vi "error_detail.vi"(10 "Error History 2":string, 11 "Device 2":string) -> ()   [LabVIEW 2020]
uses:
  Controls/comunicationQueuecluster.ctl
  Controls/PingQueueTypDef.ctl
  Controls/deviceQueue.ctl
  Controls/stopQue.ctl
  Controls/DeviceControl_Typdef.ctl
panel:
  in  "newDevice":bool=TRUE
  out "Device 3":string
  in  "Tab Control":enum32{"error", "Device", "GUI", "Computer"}(tab)=enum."Computer"
  out "Error History":string
  in  "start_device":bool=TRUE
  in  "restart_device":bool=TRUE
  in  "kill_device":bool=TRUE
  out "status:":string
  out "error:":string
  in  "Subscribed Variables":i32(listbox)
  out "response time":u32(slide) scale=0.0..5000.0
  out "devicetype:":string
  in  "start_GUI":bool=TRUE
  in  "rdp_PC":bool=TRUE
  in  "restart_PC":bool=TRUE
  out "IP":string
  in  "start_PC":bool
  in  "Cancel Button":bool
  in  "Device":bool
  in  "GUI":bool=TRUE
  in  "Computer":bool
  in  "Error":bool
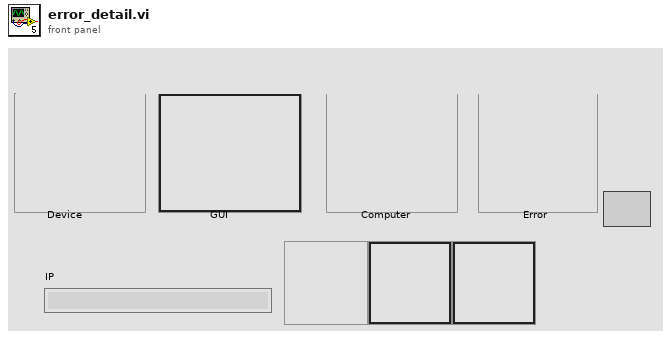
[diagram p1: front panel]
types:
  T1 = typedef "stopQue.ctl" = cluster{"stop":bool}
  T2 = enum8{"Enabled", "Disabled", "Disabled and Grayed Out"}
  T3 = typedef "deviceQueue.ctl" = cluster{"device":string[], "XY Graph":cluster{"x":u32[], "Ramp Pattern":dbl[]}, "ststus":string[], "error":string[], "error history":string[]}
  T4 = typedef "PingQueueTypDef.ctl" = cluster{"Computers not on":string[]}
  T5 = typedef "comunicationQueuecluster.ctl" = cluster{"device":string, "error history":string, "stop":bool}
  T6 = typedef "DeviceControl_Typdef.ctl" = enum16{"start", "stop", "kill", "PC rdp", "PC start", "PC shutdown", "PC restart", "GUI start"}
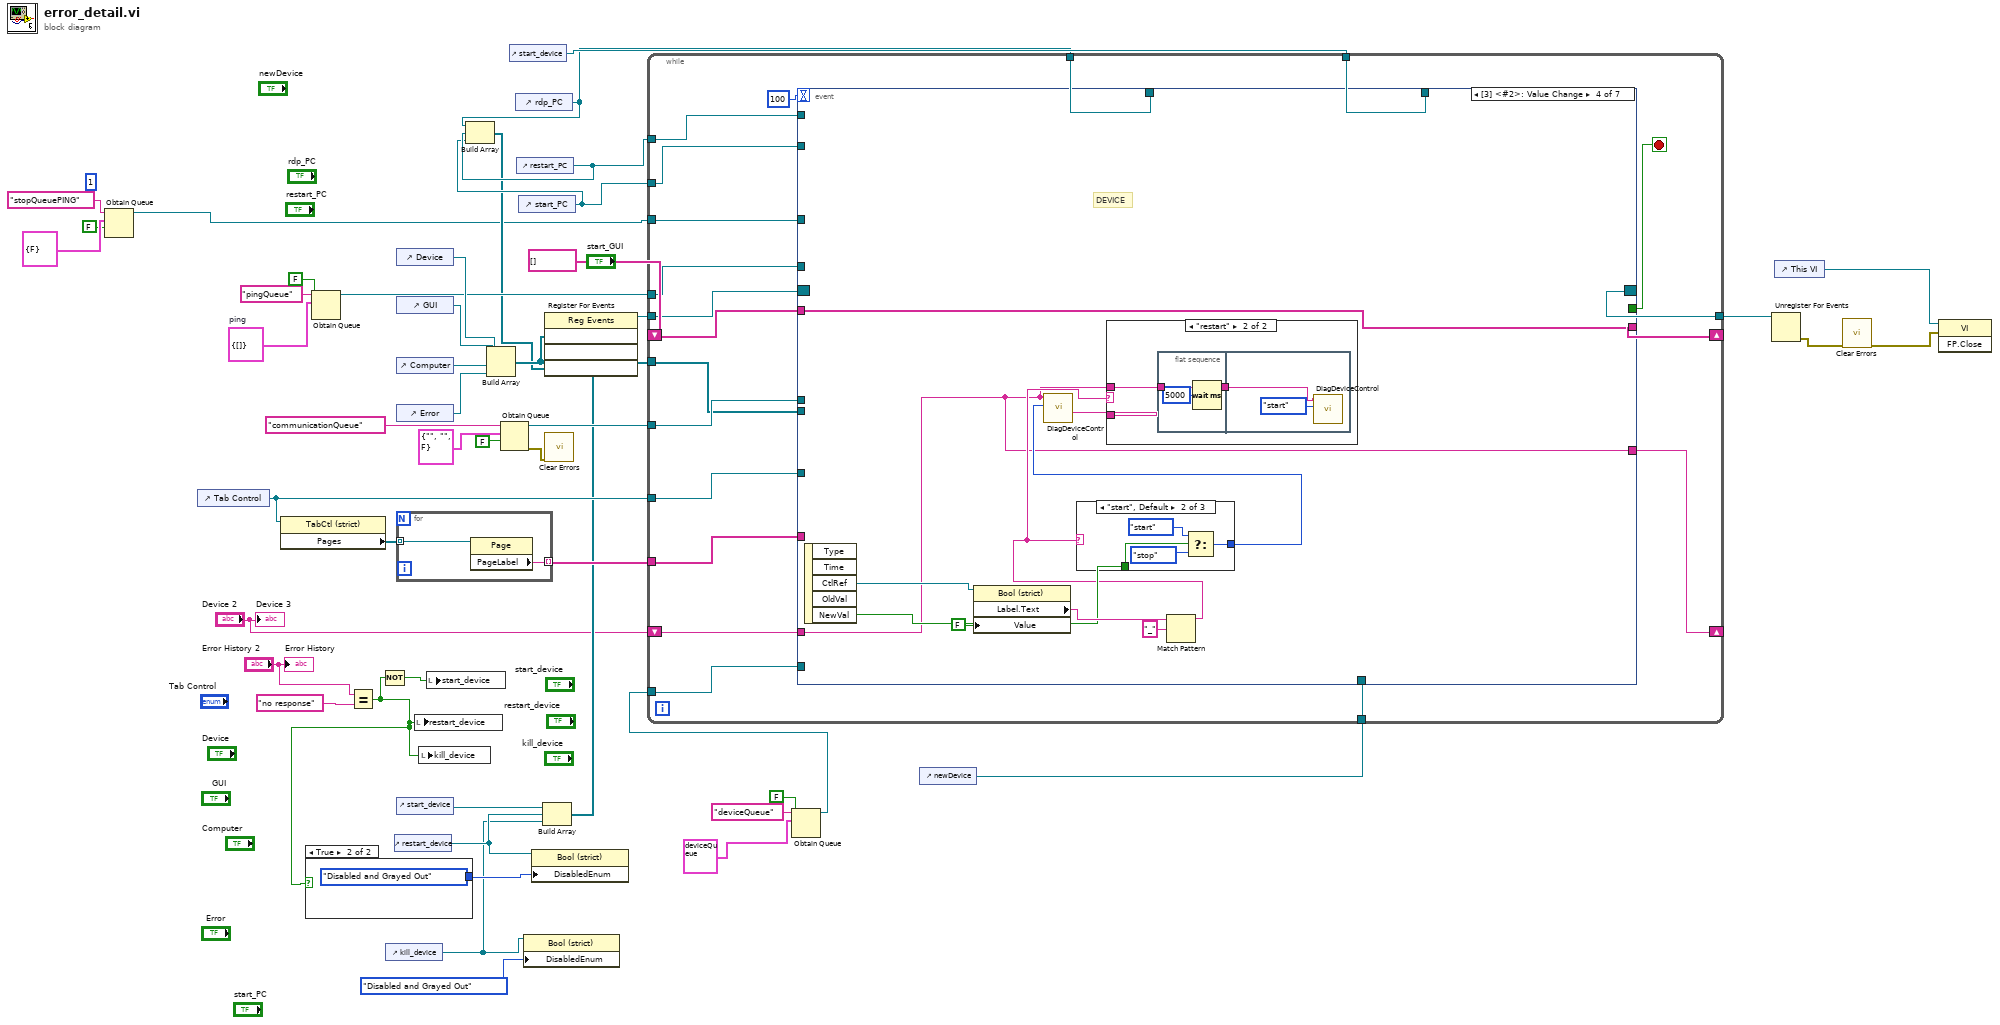
[diagram p0: block diagram]
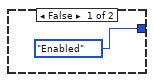
[diagram p2: hidden frame]
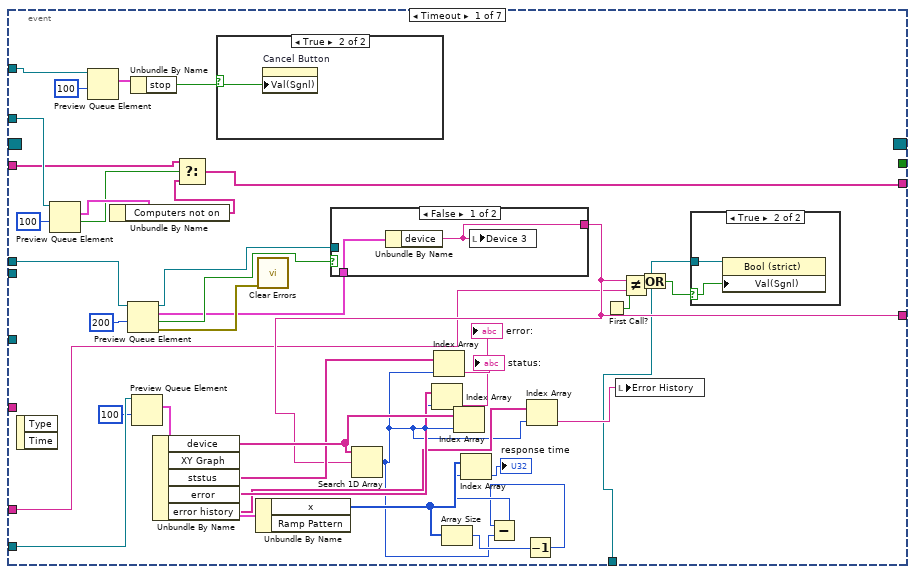
[diagram p3: hidden frame]
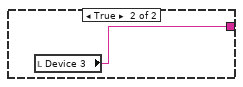
[diagram p6: hidden frame]
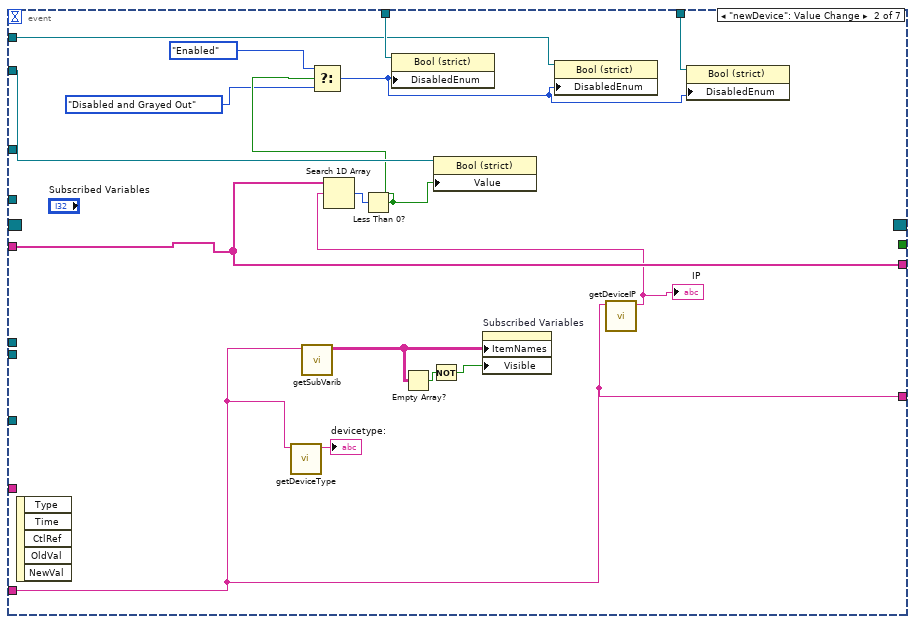
[diagram p7: hidden frame]
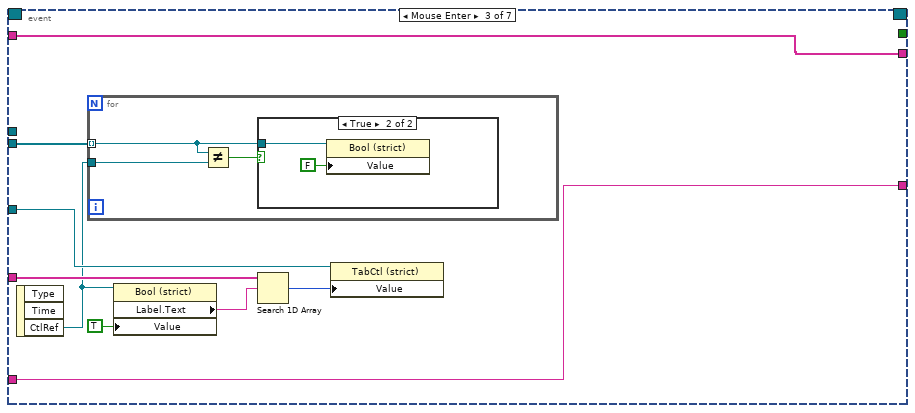
[diagram p8: hidden frame]
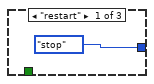
[diagram p11: hidden frame]
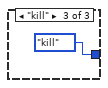
[diagram p12: hidden frame]
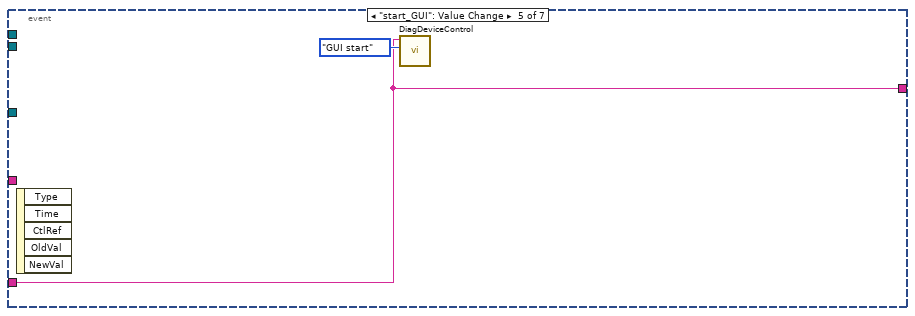
[diagram p13: hidden frame]
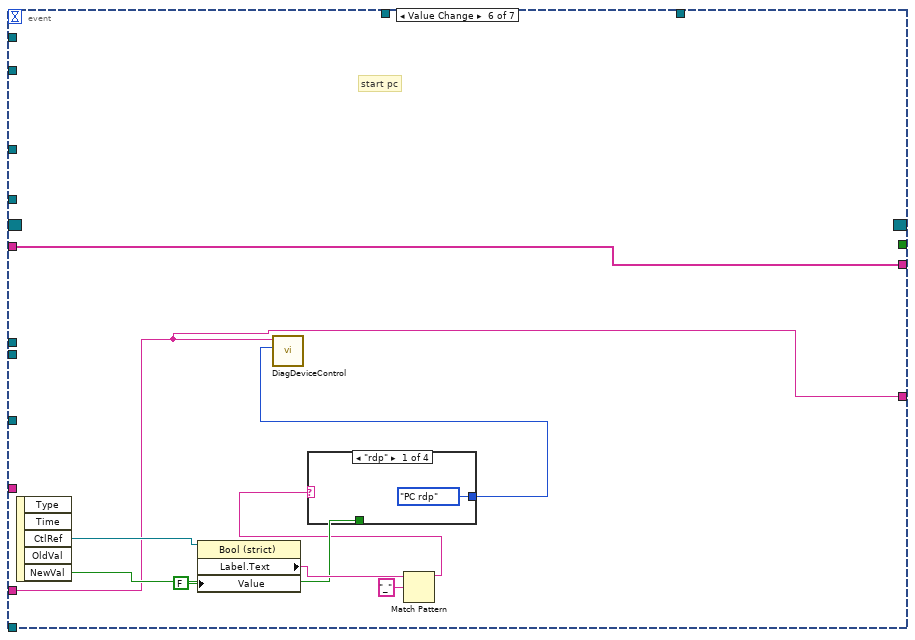
[diagram p14: hidden frame]
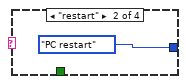
[diagram p15: hidden frame]
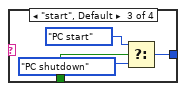
[diagram p16: hidden frame]
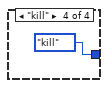
[diagram p17: hidden frame]
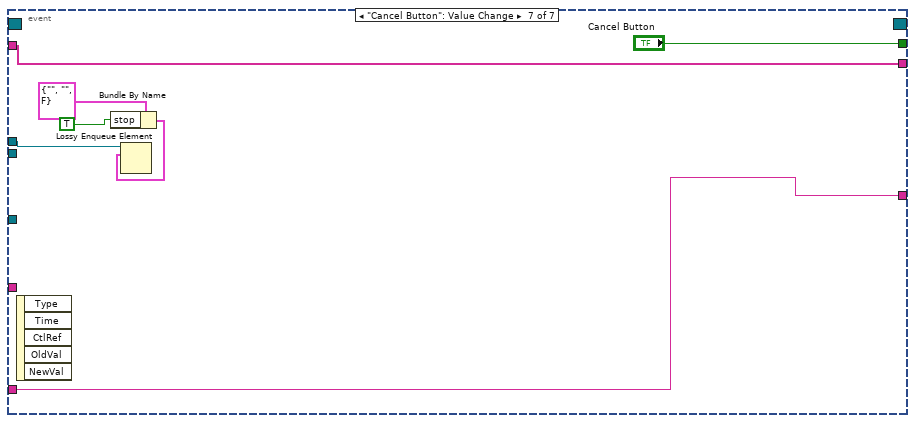
[diagram p18: hidden frame]
diagram:
  (unwired) 1 ("max queue size (-1, unlimited)")
  w22 = T4 {"Computers not on"=[]}  # ping
  n1 = Obtain Queue(name (unnamed)="stopQueuePING", element data type=T1 {"stop"=FALSE}, create if not found? (T)=FALSE) -> (queue out=w1:refnum<queue>)  [unwired: 2 in, 2 out]
  n2 = control-ref of="Tab Control"() -> (w38:refnum<vi>)
  n3 = property class="TabCtl (strict)"(reference=w38) -> ("Pages"=w37:refnum<vi>[])  [unwired: 1 in, 2 out]
  n4 = Obtain Queue(name (unnamed)="pingQueue", element data type=w22, create if not found? (T)=FALSE) -> (queue out=w15:refnum<queue>)  [unwired: 2 in, 2 out]
  n5 = Equal?(x="Error History 2", y="no response") -> (x = y?=w30:bool)
  n6 = case shown="True" w30 {
    tunnel: [T2."Enabled" ("Disabled") T2."Disabled and Grayed Out" ("Disabled")] -> w29
    frame False {
    }
    frame True {
    }
  }
  n7 = Not(x=w30) -> (.not. x?=w31:bool)
  n8 = control-ref of="kill_device"() -> (w26:refnum<vi>)
  n9 = control-ref of="restart_device"() -> (w27:refnum<vi>)
  n10 = control-ref of="Device"() -> (w44:refnum<vi>)
  n11 = control-ref of="GUI"() -> (w43:refnum<vi>)
  n12 = control-ref of="Computer"() -> (w42:refnum<vi>)
  n13 = control-ref of="Error"() -> (w41:refnum<vi>)
  n14 = for {
    tunnel: w37 -> [w52] mode=indexing
    tunnel: [w51] -> w36 mode=indexing
    n15 = property class="Page"(reference=w52) -> ("PageLabel"=w51:string)  [unwired: 1 in, 2 out]
  }
  n16 = control-ref of="start_device"() -> (w28:refnum<vi>)
  n17 = local write "restart_device"(w30) -> ()
  n18 = local write "kill_device"(w30) -> ()
  n19 = local write "start_device"(w31) -> ()
  n20 = Build Array(w44, w43, w42, w41) -> (w34:refnum<vi>[])
  n21 = Obtain Queue(name (unnamed)="communicationQueue", element data type=T5 {"device"="", "error history"="", "stop"=FALSE}, create if not found? (T)=FALSE) -> (queue out=w46:refnum<queue>, error out=w35:errorcluster)  [unwired: 2 in, 1 out]
  n22 = control-ref of="start_device"() -> (w13:refnum<vi>)
  n23 = control-ref of="rdp_PC"() -> (w12:refnum<vi>)
  n24 = control-ref of="restart_PC"() -> (w11:refnum<vi>)
  n25 = control-ref of="start_PC"() -> (w10:refnum<vi>)
  n26 = Build Array(w12, w11, w10) -> (w9:refnum<vi>[])
  n27 = property class="Bool (strict)"(reference=w26, "DisabledEnum"=T2."Disabled and Grayed Out" ("Disabled")) -> ()  [unwired: 1 in, 2 out]
  n28 = property class="Bool (strict)"(reference=w27, "DisabledEnum"=w29) -> ()  [unwired: 1 in, 2 out]
  n29 = Build Array(w28, w27, w26) -> (w25:refnum<vi>[])
  n30 = register-events(w34, w25, w9) -> (reference out=w40:refnum<event-registration>)  [unwired: 2 in, 1 out]
  n31 = call <vilib>:"Clear Errors.vi"("error in (no error)"=w35) -> ()  [unwired: 5 in, 2 out]
  n32 = Obtain Queue(name (unnamed)="deviceQueue", element data type=T3 {"device"=["StagingM1Far", "StagingM1Near", "StagingM3Far", "StagingM5", "StagingOAP2Near", "StagingOAP1Near", "StagingPXISlow", "StagingOAP2Far", "StagingLowPressure1", "StagingHexapodPI", "StagingDG645_1", "StagingLowPressure2", "StagingPXIFast2", "StagingPXIFast1", "StagingAlignBeam1", "StagingAlignBeam2", "StagingFilterWheels", "StagingShotControl", "StagingDG645_2", "StagingTRA3", "StagingGuppy", "TREX PXI fast", "StagingNISwitch", "StagingEnergy", "StagingTelescopePosition", "StagingDischargePower", "StagingDischargeHV", "StagingInterlock", "StagingAnalysisSlow", "Staging1Wire", "StagingTRA2", "StagingTelescopeImageLocation", "StagingBeam1OAPMotors", "StagingM4", "StagingDelayStage", "StagingTRA1", "StagingOAP1Far", "StagingFocusPositionBeam1", "StagingFocusPositionBeam2", "TREX TRA1", "StagingHighPressureDAQ", "StagingHighPressureController"], "XY Graph"={"x"=[154, 10000, 41, 80, 72, 7, 151, 45, 108, 239, 223, 116, 0, 109, 143, 4, 112, 224, 106, 57, 89, 58, 39, 40, 414, 148, 167, 127, 199, 314, 183, 174, 107, 5, 104, 505, 42, 76, 44, 102, 3, 30], "Ramp Pattern"=[0.0, 1.0, 2.0, 3.0, 4.0, 5.0, 6.0, 7.0, 8.0, 9.0, 10.0, 11.0, 12.0, 13.0, 14.0, 15.0, 16.0, 17.0, 18.0, 19.0, 20.0, 21.0, 22.0, 23.0, 24.0, 25.0, 26.0, 27.0, 28.0, 29.0, 30.0, 31.0, 32.0, 33.0, 34.0, 35.0, 36.0, 37.0, 38.0, 39.0, 40.0, 41.0]}, "ststus"=["Initialized", "Initialized", "Initialized", "Initialized", "Initialized", "Initialized", "Initialized", "Initialized", "Initialized", "Initialized", "Initialized", "Initialized", "Initialized", "Initialized", "Initialized", "Initialized", "Initialized", "Initialized", "Initialized", "Initialized", "Initialized", "Initialized", "Initialized", "Initialized", "Initialized", "Initialized", "Initialized", "Initialized", "Initialized", "Initialized", "Initialized", "Initialized", "Initialized", "Initialized", "Initialized", "Initialized", "Initialized", "Initialized", "Initialized", "Initialized", "no response", "Initialized"], "error"=["no error", "no error", "no error", "error", "no error", "no error", "no error", "no error", "no error", "no error", "no error", "no error", "no error", "no error", "no error", "no error", "no error", "no error", "no error", "no error", "error", "no error", "no error", "no error", "no error", "no error", "no error", "no error", "no error", "no error", "no error", "no error", "no error", "no error", "no error", "no error", "no error", "no error", "no error", "no error", "no response", "no error"], "error history"=[]} ("deviceQueue"), create if not found? (T)=FALSE) -> (queue out=w17:refnum<queue>)  [unwired: 2 in, 2 out]
  n33 = control-ref of="newDevice"() -> (w8:refnum<vi>)
  n34 = while {
    tunnel: w46 -> [w70]
    tunnel: w40 -> [w69]
    tunnel: [w68] -> w39
    tunnel: w38 -> [w67]
    tunnel: w36 -> [w66]
    tunnel: w34 -> [w65]
    tunnel: w17 -> [w63]
    tunnel: w15 -> [w62]
    tunnel: w10 -> [w61]
    tunnel: w12 -> [w60]
    tunnel: w11 -> [w59]
    shift-right: [w58] -> _
    shift-left: string[] [] ("Computers not on") -> [w57]
    tunnel: w13 -> [w56]
    shift-right: [w55] -> _
    shift-left: "Device 2" -> [w64]
    tunnel: w8 -> [w54]
    tunnel: w1 -> [w53]
    stop <- w72 stop-if-true
    n35 = event shown="[3] <#2>: Value Change" {
      selector: w69 -> [_ _ _ _ _ _ _]
      dyn-events: [_ _ _ _ _ _ _] -> w68
      timeout: 100 -> [_ _ _ _ _ _ _]
      tunnel: [_ _ _ _ _ _ "Cancel Button"] -> w72
      tunnel: w70 -> [w91 _ _ _ _ _ w192]
      tunnel: w67 -> [_ _ w143 _ _ _ _]
      tunnel: w66 -> [_ _ w142 _ _ _ _]
      tunnel: w65 -> [_ _ w139 _ _ _ _]
      tunnel: w64 -> [w81 w120 w135 w150 w171 w174 w193]
      tunnel: w63 -> [w112 _ _ _ _ _ _]
      tunnel: w62 -> [w96 _ _ _ _ _ _]
      tunnel: w61 -> [_ w133 _ _ _ _ _]
      tunnel: w60 -> [_ w129 _ _ _ _ _]
      tunnel: w59 -> [_ w128 _ _ _ _ _]
      tunnel: [w92 w125 w136 w151 _ w175 w194] -> w58
      tunnel: w57 -> [w94 w125 w136 w151 _ w175 w194]
      tunnel: w56 -> [_ w127 _ _ _ _ _]
      tunnel: [w82 w120 w135 w150 w171 w174 w193] -> w55
      tunnel: w54 -> [w80 _ _ _ _ _ _]
      tunnel: w53 -> [w75 _ _ _ _ _ _]
      event Timeout {
        n36 = event-data() -> ()  [unwired: 1 in, 2 out]
        n37 = Preview Queue Element(queue=w96, timeout in ms (-1)=100) -> (element=w97:T4, timed out?=w95:bool)  [unwired: 1 in, 2 out]
        n38 = Preview Queue Element(queue=w75, timeout in ms (-1)=100) -> (element=w74:T1)  [unwired: 1 in, 3 out]
        n39 = Unbundle By Name(w97) -> ("Computers not on"=w93:string[])
        n40 = Preview Queue Element(queue=w91, timeout in ms (-1)=200) -> (queue out=w90:refnum<queue>, element=w86:T5, timed out?=w89:bool, error out=w88:errorcluster)  [unwired: 1 in]
        n41 = Unbundle By Name(w74) -> ("stop"=w73:bool)
        n42 = Preview Queue Element(queue=w112, timeout in ms (-1)=100) -> (element=w111:T3)  [unwired: 1 in, 3 out]
        n43 = Unbundle By Name(w111) -> ("device"=w108:string[], "XY Graph"=w110:cluster{"x":u32[], "Ramp Pattern":dbl[]}, "ststus"=w102:string[], "error"=w101:string[], "error history"=w85:string[])
        n44 = Select(t=w94, s=w95, f=w93) -> (s? t:f=w92:string[])
        n45 = case shown="True" w73 {
          selector: w73 -> [_ w113]
          frame False {
          }
          frame True {
            n46 = property on="Cancel Button" class="Bool (strict)"("Val(Sgnl)"=w113) -> ()  [unwired: 2 in, 2 out]
          }
        }
        n47 = Unbundle By Name(w110) -> ("x"=w107:u32[])  [unwired: 1 out]
        n48 = call <vilib>:"Clear Errors.vi"("error in (no error)"=w88) -> ()  [unwired: 5 in, 2 out]
        n49 = case shown="False" w89 {
          tunnel: w90 -> [_ _]
          tunnel: [w116 w118] -> w82
          tunnel: w86 -> [w117 _]
          frame False {
            n50 = Unbundle By Name(w117) -> ("device"=w116:string)
            n51 = local write "Device 3"(w116) -> ()
          }
          frame True {
            n52 = local read "Device 3"() -> (w118:string)
          }
        }
        n53 = Search 1D Array(1D array=w108, element=w82) -> (index of element=w84:i32)  [unwired: 1 in]
        n54 = Index Array(array=w101, index=w84) -> (element=→"error:":string)
        n55 = Index Array(array=w102, index=w84) -> (element=→"status:":string)
        n56 = Array Size(array=w107) -> (size(s)=w104:i32)
        n57 = Index Array(array=w108, index=w84) -> ()  [unwired: 1 out]
        n58 = Decrement(x=w104) -> (x-1=w103:i32)
        n59 = Subtract(x=w103, y=w84) -> (x-y=w106:i32)
        n60 = Index Array(array=w107, index=w106) -> (element=→"response time":u32)
        n61 = Index Array(array=w85, index=w84) -> (element=w83:string)
        n62 = First Call?() -> (First Call?: T/F=w78:bool)
        n63 = local write "Error History"(w83) -> ()
        n64 = Not Equal?(x=w82, y=w81) -> (x != y?=w79:bool)
        n65 = Or(x=w79, y=w78) -> (x .or. y?=w77:bool)
        n66 = case shown="True" w77 {
          selector: w77 -> [_ w114]
          tunnel: w80 -> [_ w115]
          frame False {
          }
          frame True {
            n67 = property class="Bool (strict)"(reference=w115, "Val(Sgnl)"=w114) -> ()  [unwired: 1 in, 2 out]
          }
        }
      }
      event "newDevice": Value Change {
        n68 = event-data() -> ()  [unwired: 1 in, 5 out]
        n69 = call "getDeviceType.vi"("Device in"=w120) -> ("devicetype"=→"devicetype:":string)  [unwired: 10 in]
        n70 = call "getSubVarib.vi"("Device in"=w120) -> ("data"=w123:string[][])  [unwired: 10 in]
        n71 = Empty Array?(array=w123) -> (empty?=w122:bool)
        n72 = Not(x=w122) -> (.not. x?=w121:bool)
        n73 = property on="Subscribed Variables" class="MCListbox (strict)"("ItemNames"=w123, "Visible"=w121) -> ()  [unwired: 2 in, 2 out]
        n74 = call "getDeviceIP.vi"("Device name"=w120) -> ("userID"=w124:string)  [unwired: 10 in]
        "IP" <- w124
        n75 = Search 1D Array(1D array=w125, element=w124) -> (index of element=w134:i32)  [unwired: 1 in]
        n76 = Less Than 0?(x=w134) -> (x < 0?=w132:bool)
        n77 = Select(t=T2."Enabled" ("Disabled"), s=w132, f=T2."Disabled and Grayed Out" ("Disabled")) -> (s? t:f=w126:T2)
        n78 = property class="Bool (strict)"(reference=w129, "DisabledEnum"=w126) -> ()  [unwired: 1 in, 2 out]
        n79 = property class="Bool (strict)"(reference=w133, "Value"=w132) -> ()  [unwired: 1 in, 2 out]
        n80 = property class="Bool (strict)"(reference=w128, "DisabledEnum"=w126) -> ()  [unwired: 1 in, 2 out]
        n81 = property class="Bool (strict)"(reference=w127, "DisabledEnum"=w126) -> ()  [unwired: 1 in, 2 out]
      }
      event Mouse Enter {
        n82 = event-data() -> ("CtlRef"=w138:refnum<vi>)  [unwired: 1 in, 2 out]
        n83 = for {
          tunnel: w139 -> [w144] mode=indexing
          tunnel: w138 -> [w146]
          n84 = Not Equal?(x=w144, y=w146) -> (x != y?=w145:bool)
          n85 = case shown="True" w145 {
            tunnel: w144 -> [_ w148]
            frame False {
            }
            frame True {
              n86 = property class="Bool (strict)"(reference=w148, "Value"=FALSE) -> ()  [unwired: 1 in, 2 out]
            }
          }
        }
        n87 = property class="Bool (strict)"(reference=w138, "Value"=TRUE) -> ("Label.Text"=w141:string)  [unwired: 1 in, 2 out]
        n88 = Search 1D Array(1D array=w142, element=w141) -> (index of element=w140:i32)  [unwired: 1 in]
        n89 = property class="TabCtl (strict)"(reference=w143, "Value"=w140) -> ()  [unwired: 1 in, 2 out]
      }
      event Value Change {
        # "DEVICE"
        n90 = event-data() -> ("CtlRef"=w158:refnum<vi>, "NewVal"=w155:bool)  [unwired: 1 in, 3 out]
        n91 = property class="Bool (strict)"(reference=w158, "Value"=FALSE) -> ("Label.Text"=w157:string)  [unwired: 1 in, 2 out]
        n92 = Match Pattern(string=w157, regular expression="_") -> (before substring=w152:string)  [unwired: 1 in, 3 out]
        n93 = case shown="\"start\", Default" w152 {
          tunnel: [DeviceControl_Typdef."stop" ("Enum 2") w166 DeviceControl_Typdef."kill" ("Enum 2")] -> w154
          tunnel: w155 -> [_ w169 _]
          frame "restart" {
          }
          frame "start", Default {
            n94 = Select(t=DeviceControl_Typdef."start" ("Enum 2"), s=w169, f=DeviceControl_Typdef."stop" ("Enum 2")) -> (s? t:f=w166:T6)
          }
          frame "kill" {
          }
        }
        n95 = call "DiagDeviceControl.vi"("Enum"=w154, "Device"=w150) -> ("concatenated string"=w153:string)  [unwired: 7 in, 2 out]
        n96 = case shown="\"restart\"" w152 {
          tunnel: w153 -> [_ _]
          tunnel: w150 -> [_ w160]
          frame "False", Default {
          }
          frame "restart" {
            n97 = flat-sequence {
              tunnel: w160 -> [w162]
              tunnel: [w162] -> w159
              tunnel: w159 -> [w164]
              frame #0 {
                n98 = Wait (ms)(milliseconds to wait=u32 5000) -> ()  [unwired: 1 out]
              }
              frame #1 {
                n99 = call "DiagDeviceControl.vi"("Enum"=DeviceControl_Typdef."start", "Device"=w164) -> ()  [unwired: 7 in, 3 out]
              }
            }
          }
        }
      }
      event "start_GUI": Value Change {
        n100 = event-data() -> ()  [unwired: 1 in, 5 out]
        n101 = call "DiagDeviceControl.vi"("Enum"=DeviceControl_Typdef."GUI start", "Device"=w171) -> ()  [unwired: 7 in, 3 out]
      }
      event Value Change {
        # "start pc"
        n102 = event-data() -> ("CtlRef"=w181:refnum<vi>, "NewVal"=w178:bool)  [unwired: 1 in, 3 out]
        n103 = property class="Bool (strict)"(reference=w181, "Value"=FALSE) -> ("Label.Text"=w180:string)  [unwired: 1 in, 2 out]
        n104 = Match Pattern(string=w180, regular expression="_") -> (before substring=w176:string)  [unwired: 1 in, 3 out]
        n105 = case shown="\"rdp\"" w176 {
          tunnel: [DeviceControl_Typdef."PC rdp" ("Enum 2") DeviceControl_Typdef."PC restart" ("Enum 2") w184 DeviceControl_Typdef."kill" ("Enum 2")] -> w177
          tunnel: w178 -> [_ _ w187 _]
          frame "rdp" {
          }
          frame "restart" {
          }
          frame "start", Default {
            n106 = Select(t=DeviceControl_Typdef."PC start" ("Enum 2"), s=w187, f=DeviceControl_Typdef."PC shutdown" ("Enum 2")) -> (s? t:f=w184:T6)
          }
          frame "kill" {
          }
        }
        n107 = call "DiagDeviceControl.vi"("Enum"=w177, "Device"=w174) -> ()  [unwired: 7 in, 3 out]
      }
      event "Cancel Button": Value Change {
        n108 = event-data() -> ()  [unwired: 1 in, 5 out]
        n109 = Bundle By Name(cluster=T5 {"device"="", "error history"="", "stop"=FALSE}, "stop"=TRUE) -> (w189:T5)
        n110 = Lossy Enqueue Element(queue=w192, element=w189) -> ()  [unwired: 1 in, 4 out]
      }
    }
  }
  n111 = Unregister For Events(event registration refnum=w39) -> (error out=w7:errorcluster)  [unwired: 1 in]
  n112 = control-ref of="This VI"() -> (w5:refnum<vi>)
  n113 = call <vilib>:"Clear Errors.vi"("error in (no error)"=w7) -> ("error out"=w6:errorcluster)  [unwired: 5 in, 1 out]
  n114 = invoke class="VI" method="FP.Close"(reference=w5, error in=w6) -> ()  [unwired: 1 in, 3 out]
  "Device 3" <- "Device 2"
  "Error History" <- "Error History 2"
